vi "Read Node.vi"(8 "error in (no error)":errorcluster, 11 "abs_Decorator in":refnum<class "abs_Decorator.lvclass">) -> (0 "error out":errorcluster, 2 "BT.lvlib:abs_Node.lvclass":refnum<class "abs_Node.lvclass">, 3 "abs_Decorator out":refnum<class "abs_Decorator.lvclass">)   [LabVIEW 2021, in "BT.lvlib" / "abs_Decorator.lvclass"]
uses:
  abs_Decorator.lvclass
  abs_Node/abs_Node.lvclass
  abs_Decorator.lvclass/abs_Decorator.ctl
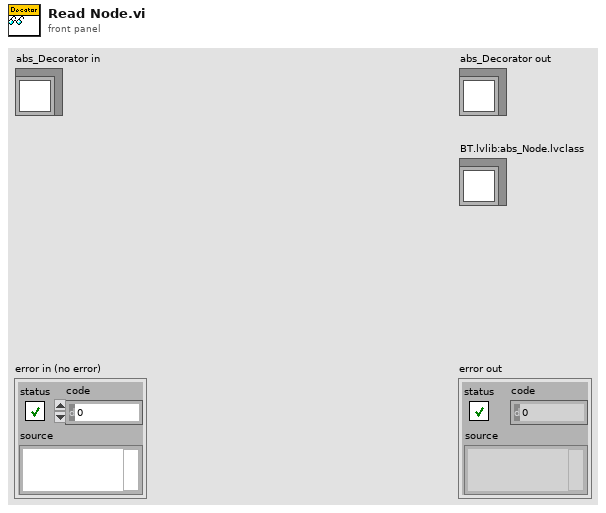
[diagram p1: front panel]
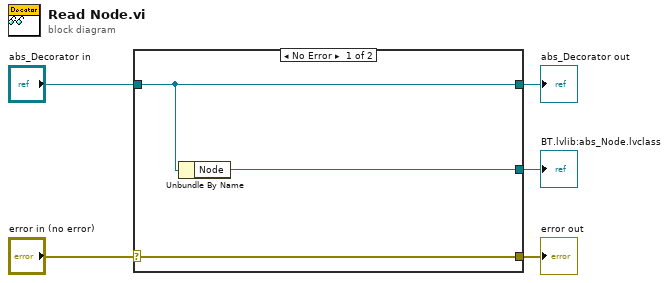
[diagram p0: block diagram]
diagram:
  n1 = case shown="No Error" "error in (no error)" {
    selector: "error in (no error)" -> [w8 w9]
    tunnel: [w8 w9] -> w4
    tunnel: [w7 w10] -> w2
    tunnel: "abs_Decorator in" -> [w7 w10]
    tunnel: [w6 _] -> w1
    frame No Error {
      n2 = Unbundle By Name(w7) -> ("Node"=w6:refnum<class "abs_Node.lvclass">)
    }
    frame Error {
    }
  }
  "error out" <- w4
  "abs_Decorator out" <- w2
  "BT.lvlib:abs_Node.lvclass" <- w1
